vi "VI Tree.vi"   [LabVIEW 2020, in "Anritsu Signal Analyzer Series.lvlib"]
doc: "This is the instrument driver for the Anritsu Signal Analyzer Series instruments. The VI Tree displays all the user-callable VIs of the instrument driver in an organized table."
uses:
  Anritsu Signal Analyzer Series.lvlib
  Configure/Measurement/Configure Spectrum Emission Mask (Measurement Setup).vi
  Configure/Configure Frequency (Start Stop).vi
  Data/Read Measurement (Adjacent Channel Power).vi
  Configure/Measurement/Configure Adjacent Channel Power (Measurement Setup).vi
  Configure/Measurement/Configure Third Order Intercept (Measurement Setup).vi
  Configure/Measurement/Configure Spurious Emission (Measurement Setup).vi
  Configure/Gate/Configure Gate View (Frequency Sweep).vi
  Data/Read Marker (All Marker).vi
panel:
  # "(c) 2014 Anritsu. ALL RIGHTS RESERVED."
  # "SEE DIAGRAM\nFOR VI TREE."
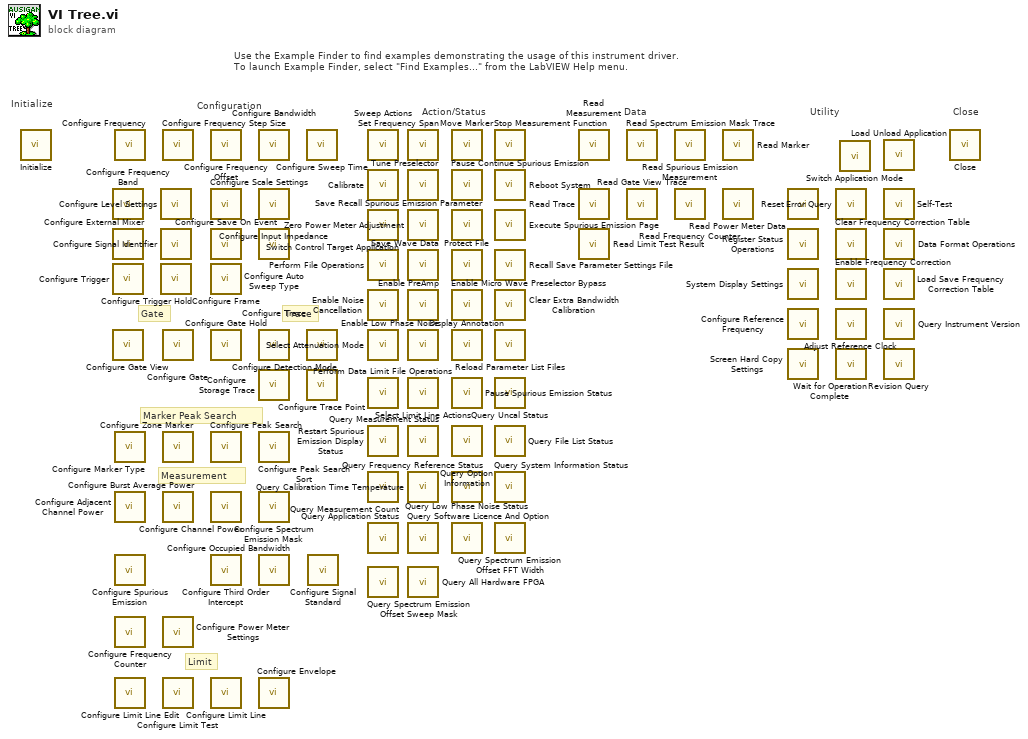
[diagram p0: block diagram]
diagram:
  # "Configuration"
  # "Utility"
  # "Data"
  # "Action/Status"
  # "Close"
  # "Initialize"
  # "Limit"
  # "Marker Peak Search"
  # "Trace"
  # "Measurement"
  # "Gate"
  # "Use the Example Finder to find examples demonstrating the usage of this instrument driver.\nTo launch Example Finder, select \"Find Examples...\" from the LabVIEW Help menu."
  n1 = call "Initialize.vi"() -> ()  [unwired: 10 in, 2 out]
  n2 = call "Configure Frequency Band.vi"() -> ()  [unwired: 14 in, 2 out]
  n3 = call "Configure External Mixer.vi"() -> ()  [unwired: 14 in, 2 out]
  n4 = call "Configure Trigger.vi"() -> ()  [unwired: 14 in, 2 out]
  n5 = call-poly "Configure Gate View.vi"() -> ()  [unwired: 14 in, 2 out]
  n6 = call-poly "Configure Frequency.vi"() -> ()  [unwired: 14 in, 2 out]
  n7 = call "Configure Marker Type.vi"() -> ()  [unwired: 14 in, 2 out]
  n8 = call-poly "Configure Adjacent Channel Power.vi"() -> ()  [unwired: 14 in, 2 out]
  n9 = call-poly "Configure Spurious Emission.vi"() -> ()  [unwired: 14 in, 2 out]
  n10 = call "Configure Frequency Counter.vi"() -> ()  [unwired: 14 in, 2 out]
  n11 = call "Configure Limit Line Edit.vi"() -> ()  [unwired: 14 in, 2 out]
  n12 = call "Configure Level Settings.vi"() -> ()  [unwired: 14 in, 2 out]
  n13 = call "Configure Signal Identifier.vi"() -> ()  [unwired: 14 in, 2 out]
  n14 = call "Configure Trigger Hold.vi"() -> ()  [unwired: 14 in, 2 out]
  n15 = call "Configure Frequency Step Size.vi"() -> ()  [unwired: 14 in, 2 out]
  n16 = call "Configure Gate.vi"() -> ()  [unwired: 14 in, 2 out]
  n17 = call "Configure Zone Marker.vi"() -> ()  [unwired: 14 in, 2 out]
  n18 = call "Configure Burst Average Power.vi"() -> ()  [unwired: 14 in, 2 out]
  n19 = call "Configure Power Meter Settings.vi"() -> ()  [unwired: 14 in, 2 out]
  n20 = call "Configure Limit Test.vi"() -> ()  [unwired: 14 in, 2 out]
  n21 = call "Configure Frequency Offset.vi"() -> ()  [unwired: 14 in, 2 out]
  n22 = call "Configure Scale Settings.vi"() -> ()  [unwired: 14 in, 2 out]
  n23 = call "Configure Save On Event.vi"() -> ()  [unwired: 14 in, 2 out]
  n24 = call "Configure Frame.vi"() -> ()  [unwired: 14 in, 2 out]
  n25 = call "Configure Gate Hold.vi"() -> ()  [unwired: 14 in, 2 out]
  n26 = call "Configure Peak Search.vi"() -> ()  [unwired: 14 in, 2 out]
  n27 = call "Configure Channel Power.vi"() -> ()  [unwired: 14 in, 2 out]
  n28 = call-poly "Configure Third Order Intercept.vi"() -> ()  [unwired: 14 in, 2 out]
  n29 = call "Configure Limit Line.vi"() -> ()  [unwired: 14 in, 2 out]
  n30 = call "Configure Bandwidth.vi"() -> ()  [unwired: 14 in, 2 out]
  n31 = call "Configure Input Impedance.vi"() -> ()  [unwired: 14 in, 2 out]
  n32 = call "Configure Auto Sweep Type.vi"() -> ()  [unwired: 14 in, 2 out]
  n33 = call "Configure Trace.vi"() -> ()  [unwired: 14 in, 2 out]
  n34 = call "Configure Storage Trace.vi"() -> ()  [unwired: 14 in, 2 out]
  n35 = call "Configure Peak Search Sort.vi"() -> ()  [unwired: 14 in, 2 out]
  n36 = call-poly "Configure Spectrum Emission Mask.vi"() -> ()  [unwired: 14 in, 2 out]
  n37 = call "Configure Occupied Bandwidth.vi"() -> ()  [unwired: 14 in, 2 out]
  n38 = call "Configure Envelope.vi"() -> ()  [unwired: 14 in, 2 out]
  n39 = call "Configure Sweep Time.vi"() -> ()  [unwired: 14 in, 2 out]
  n40 = call "Configure Detection Mode.vi"() -> ()  [unwired: 14 in, 2 out]
  n41 = call "Configure Trace Point.vi"() -> ()  [unwired: 14 in, 2 out]
  n42 = call "Configure Signal Standard.vi"() -> ()  [unwired: 14 in, 2 out]
  n43 = call "Sweep Actions.vi"() -> ()  [unwired: 14 in, 2 out]
  n44 = call "Calibrate.vi"() -> ()  [unwired: 14 in, 2 out]
  n45 = call "Switch Control Target Application.vi"() -> ()  [unwired: 14 in, 2 out]
  n46 = call "Perform File Operations.vi"() -> ()  [unwired: 14 in, 2 out]
  n47 = call "Enable Noise Cancellation.vi"() -> ()  [unwired: 14 in, 2 out]
  n48 = call "Select Attenuation Mode.vi"() -> ()  [unwired: 14 in, 2 out]
  n49 = call "Perform Data Limit File Operations.vi"() -> ()  [unwired: 14 in, 2 out]
  n50 = call "Restart Spurious Emission Display Status.vi"() -> ()  [unwired: 13 in, 3 out]
  n51 = call "Query Measurement Count.vi"() -> ()  [unwired: 13 in, 3 out]
  n52 = call "Query Application Status.vi"() -> ()  [unwired: 13 in, 3 out]
  n53 = call "Query Spectrum Emission Offset Sweep Mask.vi"() -> ()  [unwired: 13 in, 3 out]
  n54 = call "Set Frequency Span.vi"() -> ()  [unwired: 14 in, 2 out]
  n55 = call "Tune Preselector.vi"() -> ()  [unwired: 14 in, 2 out]
  n56 = call "Zero Power Meter Adjustment.vi"() -> ()  [unwired: 14 in, 2 out]
  n57 = call "Save Wave Data.vi"() -> ()  [unwired: 14 in, 2 out]
  n58 = call "Enable PreAmp.vi"() -> ()  [unwired: 14 in, 2 out]
  n59 = call "Enable Low Phase Noise.vi"() -> ()  [unwired: 14 in, 2 out]
  n60 = call "Select Limit Line Actions.vi"() -> ()  [unwired: 14 in, 2 out]
  n61 = call "Query Measurement Status.vi"() -> ()  [unwired: 13 in, 3 out]
  n62 = call "Query Calibration Time Temperature.vi"() -> ()  [unwired: 12 in, 4 out]
  n63 = call "Query Software Licence And Option.vi"() -> ()  [unwired: 11 in, 5 out]
  n64 = call "Query All Hardware FPGA.vi"() -> ()  [unwired: 13 in, 3 out]
  n65 = call "Move Marker.vi"() -> ()  [unwired: 14 in, 2 out]
  n66 = call "Pause Continue Spurious Emission .vi"() -> ()  [unwired: 14 in, 2 out]
  n67 = call "Save Recall Spurious Emission Parameter.vi"() -> ()  [unwired: 14 in, 2 out]
  n68 = call "Protect File.vi"() -> ()  [unwired: 14 in, 2 out]
  n69 = call "Enable Micro Wave Preselector Bypass.vi"() -> ()  [unwired: 14 in, 2 out]
  n70 = call "Display Annotation.vi"() -> ()  [unwired: 14 in, 2 out]
  n71 = call "Pause Spurious Emission Status.vi"() -> ()  [unwired: 13 in, 3 out]
  n72 = call "Query Option Information.vi"() -> ()  [unwired: 12 in, 4 out]
  n73 = call "Query Frequency Reference Status.vi"() -> ()  [unwired: 12 in, 4 out]
  n74 = call "Query Low Phase Noise Status.vi"() -> ()  [unwired: 13 in, 3 out]
  n75 = call "Stop Measurement Function.vi"() -> ()  [unwired: 14 in, 2 out]
  n76 = call "Reboot System.vi"() -> ()  [unwired: 14 in, 2 out]
  n77 = call "Execute Spurious Emission Page.vi"() -> ()  [unwired: 14 in, 2 out]
  n78 = call "Recall Save Parameter Settings File.vi"() -> ()  [unwired: 14 in, 2 out]
  n79 = call "Clear Extra Bandwidth Calibration.vi"() -> ()  [unwired: 14 in, 2 out]
  n80 = call "Reload Parameter List Files.vi"() -> ()  [unwired: 14 in, 2 out]
  n81 = call "Query Uncal Status.vi"() -> ()  [unwired: 13 in, 3 out]
  n82 = call "Query File List Status.vi"() -> ()  [unwired: 12 in, 4 out]
  n83 = call "Query System Information Status.vi"() -> ()  [unwired: 13 in, 3 out]
  n84 = call "Query Spectrum Emission Offset FFT Width.vi"() -> ()  [unwired: 13 in, 3 out]
  n85 = call-poly "Read Measurement.vi"() -> ()  [unwired: 13 in, 3 out]
  n86 = call "Read Trace.vi"() -> ()  [unwired: 13 in, 3 out]
  n87 = call "Read Limit Test Result.vi"() -> ()  [unwired: 13 in, 3 out]
  n88 = call "Read Spectrum Emission Mask Trace.vi"() -> ()  [unwired: 13 in, 3 out]
  n89 = call "Read Gate View Trace.vi"() -> ()  [unwired: 13 in, 3 out]
  n90 = call "Read Spurious Emission Measurement.vi"() -> ()  [unwired: 13 in, 3 out]
  n91 = call "Read Frequency Counter.vi"() -> ()  [unwired: 13 in, 3 out]
  n92 = call-poly "Read Marker.vi"() -> ()  [unwired: 13 in, 3 out]
  n93 = call "Read Power Meter Data.vi"() -> ()  [unwired: 10 in, 6 out]
  n94 = call "Reset.vi"() -> ()  [unwired: 10 in, 2 out]
  n95 = call "Register Status Operations.vi"() -> ()  [unwired: 9 in, 3 out]
  n96 = call "System Display Settings.vi"() -> ()  [unwired: 14 in, 2 out]
  n97 = call "Configure Reference Frequency.vi"() -> ()  [unwired: 14 in, 2 out]
  n98 = call "Screen Hard Copy Settings.vi"() -> ()  [unwired: 14 in, 2 out]
  n99 = call "Error Query.vi"() -> ()  [unwired: 8 in, 4 out]
  n100 = call "Clear Frequency Correction Table.vi"() -> ()  [unwired: 14 in, 2 out]
  n101 = call "Enable Frequency Correction.vi"() -> ()  [unwired: 14 in, 2 out]
  n102 = call "Adjust Reference Clock.vi"() -> ()  [unwired: 14 in, 2 out]
  n103 = call "Wait for Operation Complete.vi"() -> ()  [unwired: 10 in, 2 out]
  n104 = call "Switch Application Mode.vi"() -> ()  [unwired: 14 in, 2 out]
  n105 = call "Load Unload Application.vi"() -> ()  [unwired: 14 in, 2 out]
  n106 = call "Self-Test.vi"() -> ()  [unwired: 8 in, 4 out]
  n107 = call "Data Format Operations.vi"() -> ()  [unwired: 14 in, 2 out]
  n108 = call "Load Save Frequency Correction Table.vi"() -> ()  [unwired: 14 in, 2 out]
  n109 = call "Query Instrument Version.vi"() -> ()  [unwired: 11 in, 5 out]
  n110 = call "Revision Query.vi"() -> ()  [unwired: 9 in, 3 out]
  n111 = call "Close.vi"() -> ()  [unwired: 11 in, 1 out]
